vi "GUI_Cameras_TCP.vi"() -> ()   [LabVIEW 2013]
uses:
  <vilib>/Utility/tcp.llb/UDP Multicast Write-Only Open.vi
  <vilib>/Utility/file.llb/Read From Spreadsheet File (string).vi
  <vilib>/vision/Image Controls.llb/IMAQ Image.ctl
panel:
  out "New Image 2":T1
  in  "Device Name for vi mode":string="FakeCam1"
  out "x-y 2":u32(graph)
  out "x-y":i32(graph)
  out "x = y?":bool
  out "Numeric":i32
  out "#shot":i32=8
  out "x-y":u32(graph)
  out "data out 2":string
  out "Device Name":string="FakeCam1"
  in  "Device shotnumber":i32
  in  "New Shot":bool
  out "con ref array":refnum<vi>[](array[refnum])
  out "MC Multicast":refnum<k16>
  out "new Slow Data":bool
  out "new Device Data":bool
  in  "Tab Control":T2(tab)
  in  "setTrigger":bool
  in  "String":string="ScanStart>>Cam1only.txt"
  in  "send":bool
  in  "setSave":bool
  out "save":bool
  in  "setExposure":dbl=0.32000000000000006
  out "exposure":dbl=0.32
  out "trigger":bool=TRUE
  out "gain":dbl=10.0
  in  "setGain":dbl
  out "error message":string
  out "error":bool
  out "data out":string="Cam1>>ScanStart>>no error,>>"
  out "New Image":T1(plugin-control)
  in  "reset":bool
  in  "ScanEnd":bool
  in  "ScanStart":bool
  out "local Port":u16=64444
  out "Remote Host":string="192.168.10.157"
  out "port or service name":u16=65400
  in  "timeout ms (100)":i32=500
  in  "Multicast":bool=TRUE
  out "image \nconnection":bool
  out "data\nconnection":bool
  out "image con closed":bool=TRUE
  out "data con closed":bool=TRUE
  out "fast ID":refnum<k16>
  out "slow ID":refnum<k16>
  out "error out":errorcluster
  out "image connection ID":refnum<k5>
  out "data connection ID":refnum<k5>
  out "connections":variant[](array[variant])=[variant(refnum<k16> refnum), variant(refnum<k16> refnum)]
  in  "time to wait":i32=10
  in  "milliseconds to wait":u32=25
  in  "Image Subscriber list":string="wait>>image"
  in  "Subscriber list 2":string="wait>>exposure,trigger,save,gain"
  in  "Data String":string="exposure,0.320000\r\ntrigger,on\r\nsave,off\r\ngain,10.000000\r\n"
  out "Image":u8[][](graph)
  out "all rows":string[][](array[string])=[["localport", "64444"], ["port", "65400"], ["remotehost", "192.168.10.157"]]
  out "path":path=path "X:/Software/LOASIS Control System/Developers Version/Interface/GUI_Cameras/192.168.10.153.txt"
  out "My IP":string="192.168.10.153"
  in  "stop":bool
  # "61525"
  # "65535"
  # "61533"
  # "localhost"
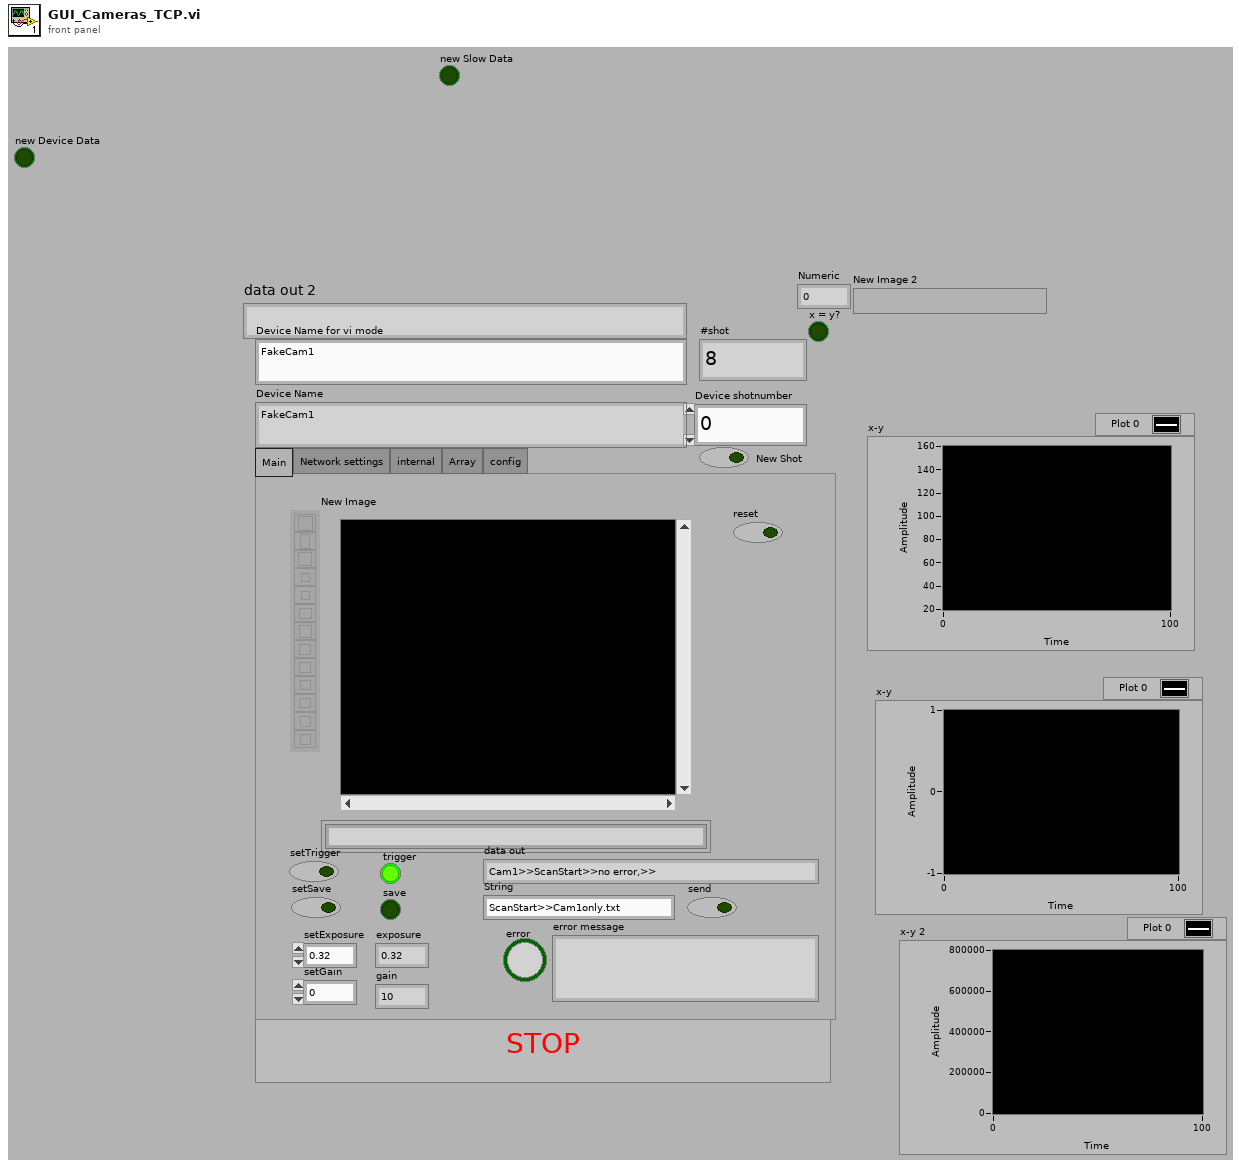
[diagram p1: front panel]
types:
  T1 = typedef "IMAQ Image.ctl" = refnum<image>
  T2 = enum32{"Main", "Network settings", "internal", "Array", "config"}
  T3 = typedef "Image Type" = u32
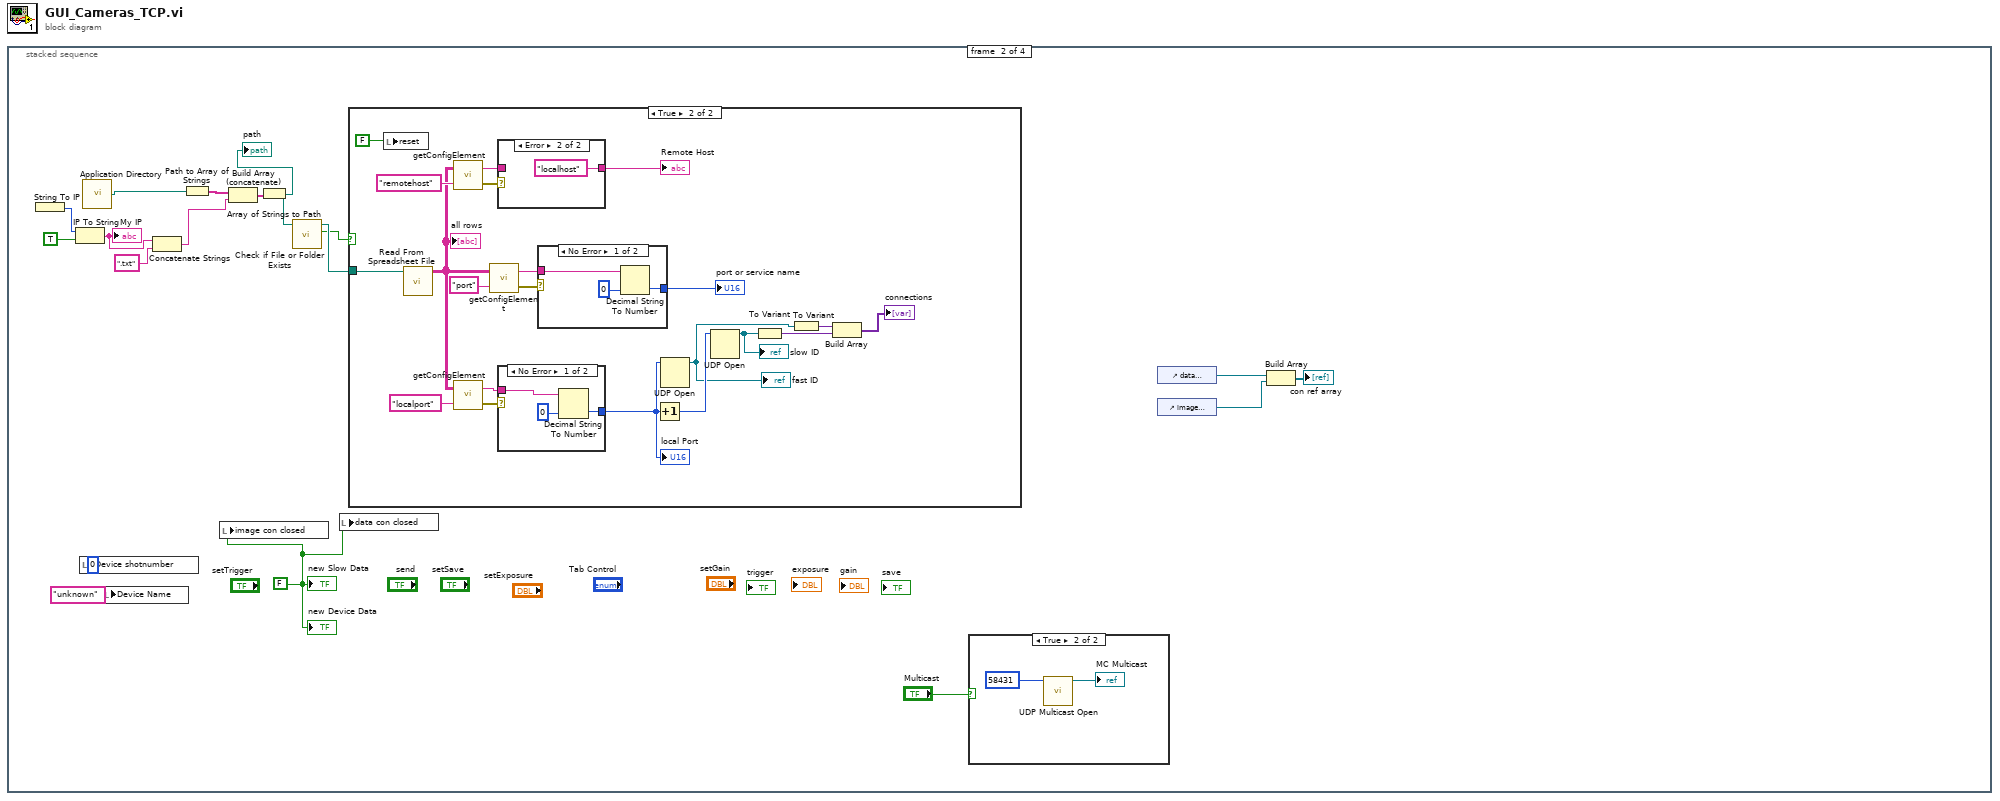
[diagram p0: block diagram]
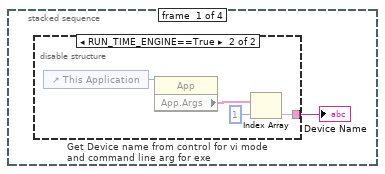
[diagram p2: hidden frame]
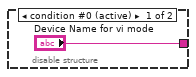
[diagram p3: hidden frame]
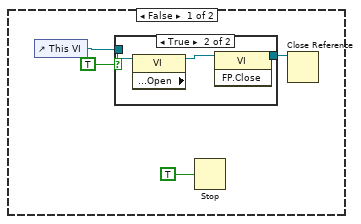
[diagram p4: hidden frame]
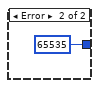
[diagram p6: hidden frame]
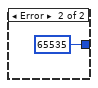
[diagram p8: hidden frame]
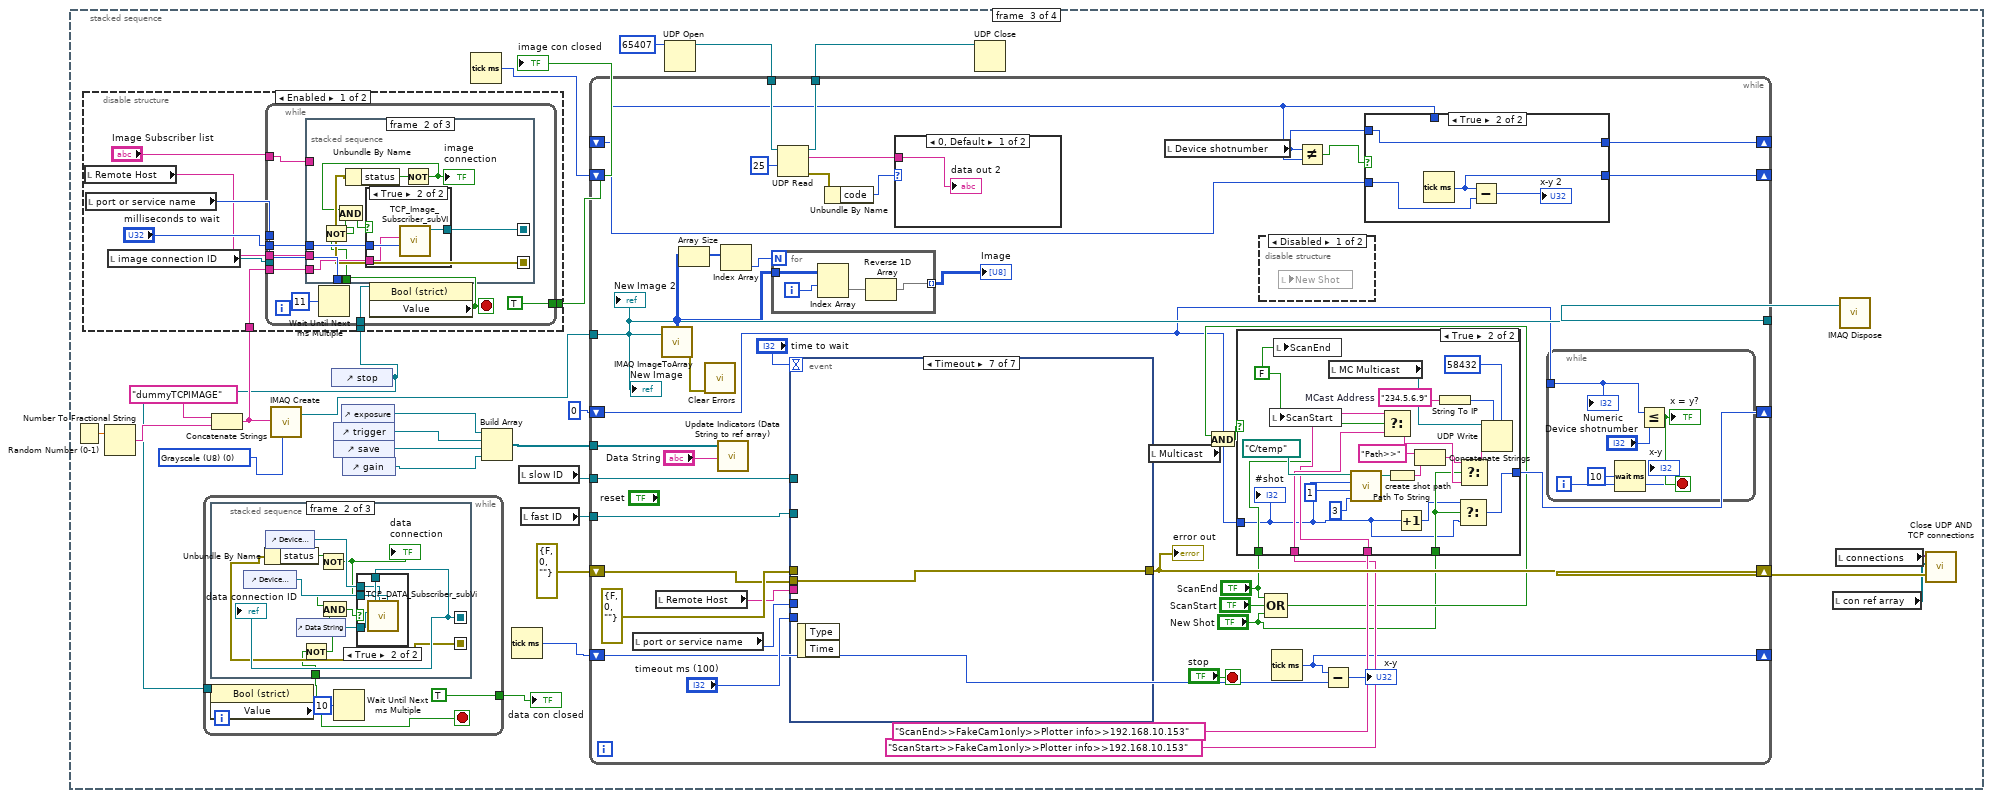
[diagram p10: hidden frame]
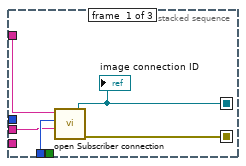
[diagram p11: hidden frame]
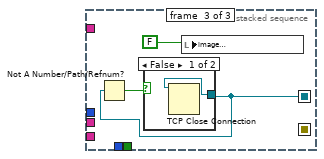
[diagram p13: hidden frame]
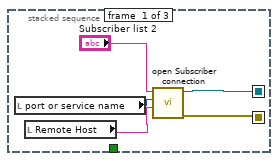
[diagram p16: hidden frame]
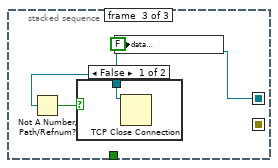
[diagram p18: hidden frame]
diagram:
  n1 = stacked-sequence {
    frame #0 {
      n2 = disable-structure "Get Device name from control for vi mode\nand command line arg for exe" shown="RUN_TIME_ENGINE==True" {
        disable-tunnel: ["Device Name for vi mode" w3] -> w1
        frame condition #0 (active) {
        }
        frame condition #1 {
          n3 = control-ref of="This Application"() -> (w6:refnum<vi>)
          n4 = property class="App"(reference=w6) -> ("App.Args"=w5:string[])  [unwired: 1 in, 2 out]
          n5 = Index Array(array=w5, index=1) -> (element=w3:string)
        }
      }
      "Device Name" <- w1
    }
    frame #1 {
      w7 = FALSE ("new Device Data")
      n6 = String To IP() -> (0:w16:u32)  [unwired: 1 in]
      n7 = IP To String(1:TRUE ("dot notation? (F)"), 2:w16) -> (0:w14:string)
      "My IP" <- w14
      n8 = local write "Device shotnumber"(0 ("shotnumber")) -> ()
      n9 = call <vilib>:"Application Directory.vi"() -> ("Application Directory"=w12:path)
      n10 = local write "Device Name"("unknown" ("Device Name")) -> ()
      n11 = Concatenate Strings(w14, ".txt" ("pattern")) -> (w11:string)
      n12 = Path to Array of Strings(0:w12) -> (2:w18:string[])  [unwired: 1 out]
      n13 = local write "image con closed"(w7) -> ()
      n14 = Build Array (concatenate)(w18, w11) -> (w17:string[])
      n15 = Array of Strings to Path(0:w17) -> (2:w10:path)  [unwired: 1 in]
      "path" <- w10
      n16 = call <vilib>:"Check if File or Folder Exists.vi"("path"=w10) -> ("file or folder exists?"=w8:bool, "dup path"=w9:path)  [unwired: 8 in, 1 out]
      n17 = local write "data con closed"(w7) -> ()
      n18 = case shown="True" w8 {
        tunnel: w9 -> [_ w33]
        frame False {
          n19 = control-ref of="This VI"() -> (w27:refnum<vi>)
          n20 = case shown="True" TRUE {
            tunnel: w27 -> [w29 w32]
            tunnel: [w29 w30] -> w26
            frame False {
            }
            frame True {
              n21 = property class="VI" props=["Front Panel.Open"](reference=w32) -> (reference out=w31:refnum<vi>)  [unwired: 1 in, 2 out]
              n22 = invoke class="VI" method="FP.Close"(reference=w31) -> (reference out=w30:refnum<vi>)  [unwired: 2 in, 2 out]
            }
          }
          n23 = Stop(stop? (T)=TRUE) -> ()
          n24 = Close Reference(reference=w26) -> ()  [unwired: 1 in, 1 out]
        }
        frame True {
          n25 = local write "reset"(FALSE ("reset")) -> ()
          n26 = call-poly <vilib>:"Read From Spreadsheet File.vi"("file path (dialog if empty)"=w33) -> ("all rows"=w35:string[][])  [unwired: 6 in, 4 out]
          "all rows" <- w35
          n27 = call "getConfigElement.vi"("element"="remotehost", "all rows"=w35) -> ("error in"=w42:errorcluster, "value"=w41:string)
          n28 = call "getConfigElement.vi"("element"="localport", "all rows"=w35) -> ("error in"=w44:errorcluster, "value"=w45:string)
          n29 = call "getConfigElement.vi"("element"="port", "all rows"=w35) -> ("error in"=w38:errorcluster, "value"=w37:string)
          n30 = case shown="Error" w42 {
            tunnel: w41 -> [w58 _]
            tunnel: [w58 "localhost" ("value")] -> w39
            frame No Error {
            }
            frame Error {
            }
          }
          "Remote Host" <- w39
          n31 = case shown="No Error" w44 {
            tunnel: w45 -> [w62 _]
            tunnel: [w60 u16 65535] -> w43
            frame No Error {
              n32 = Decimal String To Number(string=w62, default (0L)=u16 0 ("local Port")) -> (number=w60:u16)  [unwired: 1 in, 1 out]
            }
            frame Error {
            }
          }
          "local Port" <- w43
          n33 = case shown="No Error" w38 {
            tunnel: w37 -> [w56 _]
            tunnel: [w54 u16 65535] -> w34
            frame No Error {
              n34 = Decimal String To Number(string=w56, default (0L)=u16 0 ("local Port")) -> (number=w54:u16)  [unwired: 1 in, 1 out]
            }
            frame Error {
            }
          }
          "port or service name" <- w34
          n35 = Increment(x=w43) -> (x+1=w53:u16)
          n36 = UDP Open(11:w43) -> (port=w51:refnum<k16>)  [unwired: 4 in, 2 out]
          "fast ID" <- w51
          n37 = UDP Open(11:w53) -> (port=w50:refnum<k16>)  [unwired: 4 in, 2 out]
          "slow ID" <- w50
          n38 = To Variant(anything=w50) -> (Variant=w48:variant)
          n39 = To Variant(anything=w51) -> (Variant=w49:variant)
          n40 = Build Array(w49, w48) -> (→"connections":variant[])
        }
      }
      n41 = case shown="True" "Multicast" {
        frame False {
        }
        frame True {
          n42 = call-poly <vilib>:"UDP Multicast Open.vi"("port"=u16 58431) -> ("connection ID"=→"MC Multicast":refnum<k16>)  [unwired: 9 in, 1 out]
        }
      }
      n43 = control-ref of="data connection ID"() -> (w24:refnum<vi>)
      n44 = control-ref of="image connection ID"() -> (w23:refnum<vi>)
      n45 = Build Array(w24, w23) -> (→"con ref array":refnum<vi>[])
      "new Device Data" <- w7
      "new Slow Data" <- w7
    }
    frame #2 {
      w86 = T3 0 items=["Grayscale (U8)", "Grayscale (I16)", "Grayscale (SGL)", "Complex (CSG)", "RGB (U32)", "HSL (U32)", "RGB (U64)", "Grayscale (U16)"] ("Image Type")
      n46 = Random Number (0-1)() -> (number: 0 to 1=w83:dbl)
      n47 = Number To Fractional String(number=w83) -> (F-format string=w82:string)  [unwired: 3 in]
      n48 = Concatenate Strings("dummyTCPIMAGE" ("Image Name"), w82) -> (w80:string)
      n49 = call "IMAQ Create"("Image Name"=w80, "Image Type"=w86) -> ("New Image"=w85:T1)  [unwired: 3 in, 1 out]
      n50 = control-ref of="stop"() -> (w73:refnum<vi>)
      n51 = disable-structure shown="Enabled" {
        disable-tunnel: w80 -> [w98 _]
        disable-tunnel: [w94 _] -> w75
        disable-tunnel: w73 -> [w93 _]
        frame Enabled {
          n52 = local read "Remote Host"() -> (w96:string)
          n53 = local read "port or service name"() -> (w97:u16)
          n54 = local read "image connection ID"() -> (w100:refnum<k5>)
          n55 = while {
            tunnel: w100 -> [_]
            tunnel: "milliseconds to wait" -> [w109]
            tunnel: w98 -> [w108]
            tunnel: w97 -> [w107]
            tunnel: w96 -> [w106]
            tunnel: "Image Subscriber list" -> [w105]
            tunnel: [TRUE] -> w94
            tunnel: w93 -> [w102]
            stop <- w101 stop-if-true
            n56 = Wait Until Next ms Multiple(millisecond multiple=u32 11) -> ()  [unwired: 1 out]
            n57 = property class="Bool (strict)"(reference=w102) -> ("Value"=w101:bool)  [unwired: 1 in, 2 out]
            n58 = stacked-sequence {
              seq-local: [w112 _ _] -> [_ w121 w128]
              seq-local: [w110 _ _] -> [_ w120 _]
              tunnel: w109 -> [_ w123 _]
              tunnel: w108 -> [_ w122 _]
              tunnel: w107 -> [w114 _ _]
              tunnel: w106 -> [w113 _ _]
              tunnel: w105 -> [w111 _ _]
              tunnel: w101 -> [_ w118 _]
              frame #0 {
                n59 = call "open Subscriber connection.vi"("Machine"=w113, "Port"=w114, "Subscriber list"=w111) -> ("error out"=w110:errorcluster, "connection ID"=w112:refnum<k5>)  [unwired: 3 in]
                "image connection ID" <- w112
              }
              frame #1 {
                n60 = Not(x=w118) -> (.not. x?=w117:bool)
                n61 = Unbundle By Name(w120) -> ("status"=w119:bool)
                n62 = Not(x=w119) -> (.not. x?=w116:bool)
                "image \nconnection" <- w116
                n63 = And(x=w116, y=w117) -> (x .and. y?=w115:bool)
                n64 = case shown="True" w115 {
                  tunnel: w123 -> [_ w126]
                  tunnel: w122 -> [_ w125]
                  tunnel: w121 -> [_ w124]
                  frame False {
                  }
                  frame True {
                    n65 = call "TCP_Image_Subscriber_subVI.vi"(9:w126, "Image Name"=w125, "connection ID"=w124) -> ()  [unwired: 8 in, 1 out]
                  }
                }
              }
              frame #2 {
                n66 = Not A Number/Path/Refnum?(number/path/refnum=w128) -> (NaN/Path/Refnum?=w129:bool)
                n67 = case shown="False" w129 {
                  tunnel: w128 -> [w130 _]
                  frame False {
                    n68 = TCP Close Connection(connection ID=w130) -> ()  [unwired: 2 in, 2 out]
                  }
                  frame True {
                  }
                }
                n69 = local write "image \nconnection"(FALSE ("status")) -> ()
              }
            }
          }
        }
        frame Disabled {
        }
      }
      "image con closed" <- w75
      n70 = while {
        tunnel: [TRUE] -> w74
        tunnel: w73 -> [w132]
        stop <- w131 stop-if-true
        n71 = property class="Bool (strict)"(reference=w132) -> ("Value"=w131:bool)  [unwired: 1 in, 2 out]
        n72 = stacked-sequence {
          seq-local: [w136 _ _] -> [_ w148 w155]
          seq-local: [w135 _ _] -> [_ w147 _]
          tunnel: w131 -> [_ w141 _]
          frame #0 {
            n73 = local read "port or service name"() -> (w138:u16)
            n74 = local read "Remote Host"() -> (w137:string)
            n75 = call "open Subscriber connection.vi"("Machine"=w137, "Port"=w138, "Subscriber list"="Subscriber list 2") -> ("error out"=w135:errorcluster, "connection ID"=w136:refnum<k5>)  [unwired: 3 in]
          }
          frame #1 {
            n76 = control-ref of="Device shotnumber"() -> (w146:refnum<vi>)
            n77 = Unbundle By Name(w147) -> ("status"=w144:bool)
            n78 = control-ref of="Device Name"() -> (w145:refnum<vi>)
            n79 = control-ref of="Data String"() -> (w149:refnum<vi>)
            n80 = Not(x=w141) -> (.not. x?=w142:bool)
            n81 = Not(x=w144) -> (.not. x?=w143:bool)
            "data\nconnection" <- w143
            n82 = And(x=w143, y=w142) -> (x .and. y?=w140:bool)
            n83 = case shown="True" w140 {
              tunnel: w149 -> [_ w153]
              tunnel: w148 -> [_ w152]
              tunnel: w146 -> [_ w151]
              tunnel: w145 -> [_ w150]
              frame False {
              }
              frame True {
                n84 = call "TCP_DATA_Subscriber_subVi.vi"("shot number"=w151, "whatamI"=w150, 10:w153, "connection ID"=w152) -> ()  [unwired: 7 in, 1 out]
              }
            }
            "data connection ID" <- w148
          }
          frame #2 {
            n85 = Not A Number/Path/Refnum?(number/path/refnum=w155) -> (NaN/Path/Refnum?=w156:bool)
            n86 = case shown="False" w156 {
              tunnel: w155 -> [w157 _]
              frame False {
                n87 = TCP Close Connection(connection ID=w157) -> ()  [unwired: 2 in, 2 out]
              }
              frame True {
              }
            }
            n88 = local write "data\nconnection"(FALSE ("status 2")) -> ()
          }
        }
        n89 = Wait Until Next ms Multiple(millisecond multiple=u32 10) -> ()  [unwired: 1 out]
      }
      "data con closed" <- w74
      n90 = control-ref of="trigger"() -> (w87:refnum<vi>)
      n91 = control-ref of="save"() -> (w71:refnum<vi>)
      n92 = control-ref of="exposure"() -> (w88:refnum<vi>)
      n93 = control-ref of="gain"() -> (w72:refnum<vi>)
      n94 = Tick Count (ms)() -> (millisecond timer value=w66:u32)
      n95 = Build Array(w88, w87, w71, w72) -> (w79:refnum<vi>[])
      n96 = Tick Count (ms)() -> (millisecond timer value=w67:u32)
      n97 = local read "slow ID"() -> (w90:refnum<k16>)
      n98 = local read "fast ID"() -> (w91:refnum<k16>)
      n99 = UDP Open(11:u16 65407 ("port")) -> (port=w69:refnum<k16>)  [unwired: 4 in, 2 out]
      n100 = while {
        tunnel: w91 -> [w191]
        shift-right: [w189] -> w84
        shift-left: errorcluster {"status"=FALSE, "code"=0, "source"=""} ("error out") -> [w195]
        tunnel: w90 -> [w185]
        tunnel: w85 -> [w198]
        tunnel: [w198] -> w89
        tunnel: w79 -> [w197]
        shift-right: [w188] -> _
        shift-left: 0 -> [w164]
        tunnel: w69 -> [w178]
        tunnel: [w177] -> w68
        shift-right: [w166] -> _
        shift-left: w67 -> [w167]
        shift-right: [w161] -> _
        shift-left: _ -> [w158]
        shift-right: [w159] -> _
        shift-left: w66 -> [w160]
        stop <- "stop" stop-if-true
        n101 = local read "port or service name"() -> (w192:u16)
        n102 = local read "Remote Host"() -> (w193:string)
        n103 = call "IMAQ ImageToArray"("Image"=w198) -> ("error out"=w184:errorcluster, "Image Pixels (U8)"=w181:u8[][])  [unwired: 3 in, 3 out]
        n104 = Array Size(array=w181) -> (size(s)=w183:i32[])
        n105 = call <vilib>:"Clear Errors.vi"("error in (no error)"=w184) -> ()  [unwired: 6 in, 1 out]
        n106 = call "Update Indicators (Data String to ref array).vi"("Data String"="Data String", "Array"=w197) -> ()  [unwired: 4 in]
        n107 = Index Array(array=w183) -> (element=w182:i32)  [unwired: 1 in]
        n108 = for {
          N: w182 -> [_]
          tunnel: w181 -> [w216]
          tunnel: [w214] -> w180 mode=indexing
          i -> [w213]
          n109 = Index Array(array=w216, index (row)=w213) -> (element=w215:u8[])  [unwired: 1 in]
          n110 = Reverse 1D Array(array=w215) -> (reversed array=w214:u8[])
        }
        "Image" <- w180
        n111 = UDP Read(connection ID=w178, timeout ms (25000)=25) -> (data out=w173:string, error out=w175:errorcluster, 3:w177:refnum<k16>)  [unwired: 2 in, 2 out]
        n112 = event shown="[6] Timeout" {
          selector: _ -> [_ _ _ _ _ _ _]
          dyn-events: _ -> [_ _ _ _ _ _ _]
          timeout: "time to wait" -> [_ _ _ _ _ _ _]
          tunnel: w191 -> [w243 w261 _ w277 w290 w306 _]
          tunnel: [w241 w259 _ w275 w287 w304 w310] -> w189
          tunnel: errorcluster {"status"=FALSE, "code"=0, "source"=""} ("error out") -> [w242 w260 _ w276 w288 w305 _]
          tunnel: w193 -> [w246 w258 _ w274 w291 w303 _]
          tunnel: w192 -> [w247 w257 _ w273 w286 w302 _]
          tunnel: "timeout ms (100)" -> [w248 w256 _ w272 w285 w301 _]
          tunnel: w185 -> [w244 w262 _ w278 w289 w307 _]
          tunnel: w195 -> [_ _ _ _ _ _ w310]
          event "setTrigger": Value Change {
            n113 = event-data() -> ("NewVal"=w253:bool)  [unwired: 1 in, 4 out]
            n114 = Select(t="on", s=w253, f="off") -> (s? t:f=w249:string)
            n115 = Concatenate Strings("settrigger>>" ("data in"), w249) -> (w245:string)
            n116 = call "sendCommandAndListen.vi"(0:w244, 1:w243, "command in"=w245, "error in"=w242, "Remote Host"=w246, "port or service name"=w247, "timeout ms (100)"=w248) -> ("error"=w239:bool, "error message"=w240:string, "error out"=w241:errorcluster)  [unwired: 5 in, 5 out]
            n117 = local write "error message"(w240) -> ()
            n118 = local write "error"(w239) -> ()
          }
          event "setExposure": Value Change {
            n119 = event-data() -> ("NewVal"=w264:dbl)  [unwired: 1 in, 4 out]
            n120 = Number To Fractional String(number=w264) -> (F-format string=w265:string)  [unwired: 3 in]
            n121 = Concatenate Strings("setexposure>>" ("data in"), w265) -> (w263:string)
            n122 = call "sendCommandAndListen.vi"(0:w262, 1:w261, "command in"=w263, "error in"=w260, "Remote Host"=w258, "port or service name"=w257, "timeout ms (100)"=w256) -> ("error"=→"error":bool, "error message"=→"error message":string, "error out"=w259:errorcluster)  [unwired: 5 in, 5 out]
          }
          event "reset": Value Change {
            n123 = event-data() -> ()  [unwired: 1 in, 5 out]
            n124 = local read "con ref array"() -> (w268:refnum<vi>[])
            n125 = local write "Device Name"("unknown" ("Device Name")) -> ()
            n126 = local write "reset"(FALSE ("reset")) -> ()
            n127 = call "Close UDP AND TCP connections.vi"("appended array 2"=w268) -> ()  [unwired: 7 in]
          }
          event "setGain": Value Change {
            n128 = event-data() -> ("NewVal"=w280:dbl)  [unwired: 1 in, 4 out]
            n129 = Number To Fractional String(number=w280) -> (F-format string=w281:string)  [unwired: 3 in]
            n130 = Concatenate Strings("setgain>>" ("data in"), w281) -> (w279:string)
            n131 = call "sendCommandAndListen.vi"(0:w278, 1:w277, "command in"=w279, "error in"=w276, "Remote Host"=w274, "port or service name"=w273, "timeout ms (100)"=w272) -> ("error"=w270:bool, "error message"=w271:string, "error out"=w275:errorcluster)  [unwired: 5 in, 5 out]
            n132 = local write "error message"(w271) -> ()
            n133 = local write "error"(w270) -> ()
          }
          event "setSave": Value Change {
            n134 = event-data() -> ("NewVal"=w297:bool)  [unwired: 1 in, 4 out]
            n135 = Select(t="on", s=w297, f="off") -> (s? t:f=w293:string)
            n136 = Concatenate Strings("setsave>>" ("data in"), w293) -> (w292:string)
            n137 = call "sendCommandAndListen.vi"(0:w289, 1:w290, "command in"=w292, "error in"=w288, "Remote Host"=w291, "port or service name"=w286, "timeout ms (100)"=w285) -> ("error"=w283:bool, "error message"=w284:string, "error out"=w287:errorcluster)  [unwired: 5 in, 5 out]
            n138 = local write "error message"(w284) -> ()
            n139 = local write "error"(w283) -> ()
          }
          event "send": Value Change {
            n140 = event-data() -> ()  [unwired: 1 in, 5 out]
            n141 = local write "send"(FALSE ("sent")) -> ()
            n142 = call "sendCommandAndListen.vi"(0:w307, 1:w306, "command in"="String", "error in"=w305, "Remote Host"=w303, "port or service name"=w302, "timeout ms (100)"=w301) -> ("error"=w299:bool, "error message"=w300:string, "data out"=→"data out":string, "error out"=w304:errorcluster)  [unwired: 5 in, 4 out]
            n143 = local write "error message"(w300) -> ()
            n144 = local write "error"(w299) -> ()
          }
          event Timeout {
            n145 = event-data() -> ()  [unwired: 1 in, 2 out]
          }
        }
        "error out" <- w189
        n146 = Unbundle By Name(w175) -> ("code"=w174:i32)
        n147 = case shown="0, Default" w174 {
          tunnel: w173 -> [w212 _]
          frame 0, Default {
            "data out 2" <- w212
          }
          frame 56 {
          }
        }
        n148 = local read "Multicast"() -> (w187:bool)
        n149 = local read "Device shotnumber"() -> (w162:i32)
        n150 = disable-structure shown="Disabled" {
          frame Disabled {
            n151 = local read "New Shot"() -> ()  [unwired: 1 in]
          }
          frame Enabled {
          }
        }
        n152 = Compound Arithmetic op=OR("ScanEnd", "ScanStart", "New Shot") -> (w170:bool)
        n153 = And(x=w170, y=w187) -> (x .and. y?=w186:bool)
        n154 = case shown="True" w186 {
          tunnel: w164 -> [w217 w219]
          tunnel: [w217 w218] -> w188
          tunnel: "New Shot" -> [_ w221]
          tunnel: "ScanEnd>>FakeCam1only>>Plotter info>>192.168.10.153" ("String 2") -> [_ w226]
          tunnel: "ScanStart>>FakeCam1only>>Plotter info>>192.168.10.153" ("String 3") -> [_ w227]
          tunnel: "ScanEnd" -> [_ w223]
          frame False {
          }
          frame True {
            w222 = FALSE ("New Shot")
            w232 = "234.5.6.9"  # MCast Address
            n155 = local write "ScanStart"(w222) -> ()
            n156 = local write "ScanEnd"(w222) -> ()
            n157 = local read "MC Multicast"() -> (w233:refnum<k16>)
            n158 = call "create shot path.vi"("width (-)"=i16 3, "Shot Number"=w219, "Scan Number"=1, "Scans Path"=path "C:/temp") -> ("Device xxx path"=w236:path)  [unwired: 2 in]
            n159 = Select(t=w226, s=w223, f=w227) -> (s? t:f=w225:string)
            n160 = Path To String(path=w236) -> (string=w234:string)
            n161 = Increment(x=w219) -> (x+1=w220:i32)
            n162 = Concatenate Strings("Path>>" ("string"), w234) -> (w224:string)
            n163 = String To IP(1:w232) -> (0:w238:u32)
            n164 = Select(t=w220, s=w221, f=w219) -> (s? t:f=w218:i32)
            n165 = Select(t=w224, s=w221, f=w225) -> (s? t:f=w228:string)
            n166 = UDP Write(address=w238, port or service name=u16 58432, connection ID=w233, data in=w228) -> ()  [unwired: 2 in, 2 out]
            "#shot" <- w219
          }
        }
        n167 = Tick Count (ms)() -> (millisecond timer value=w166:u32)
        n168 = Not Equal?(x=w162, y=w158) -> (x != y?=w163:bool)
        n169 = Subtract(x=w166, y=w167) -> (x-y=→"x-y":u32)
        n170 = case shown="True" w163 {
          tunnel: w162 -> [_ w206]
          tunnel: [w202 w206] -> w161
          tunnel: w158 -> [w202 _]
          tunnel: w160 -> [w201 w205]
          tunnel: [w201 w204] -> w159
          frame False {
          }
          frame True {
            n171 = Tick Count (ms)() -> (millisecond timer value=w204:u32)
            n172 = Subtract(x=w204, y=w205) -> (x-y=→"x-y 2":u32)
          }
        }
        n173 = while {
          tunnel: w164 -> [w210]
          i -> [w207]
          stop <- w208 stop-if-true
          n174 = Wait (ms)(milliseconds to wait=u32 10) -> ()  [unwired: 1 out]
          n175 = Less Or Equal?(x=w210, y="Device shotnumber") -> (x <= y?=w208:bool)
          "x = y?" <- w208
          "Numeric" <- w210
          "x-y" <- w207
        }
        "New Image" <- w198
        "New Image 2" <- w198
      }
      n176 = UDP Close(connection ID=w68) -> ()  [unwired: 1 in, 2 out]
      n177 = local read "con ref array"() -> (w78:refnum<vi>[])
      n178 = local read "connections"() -> (w76:variant[])
      n179 = call "IMAQ Dispose"("Image"=w89) -> ()  [unwired: 5 in, 1 out]
      n180 = call "Close UDP AND TCP connections.vi"("error in"=w84, "appended array 2"=w78, "appended array"=w76) -> ()  [unwired: 5 in]
    }
    frame #3 {
      n181 = flat-sequence {
        frame #0 {
          n182 = Wait (ms)(milliseconds to wait=u32 0) -> ()  [unwired: 1 out]
        }
        frame #1 {
          n183 = local write "stop"(FALSE ("stop")) -> ()
        }
        frame #2 {
          n184 = control-ref of="This VI"() -> (w315:refnum<vi>)
          n185 = case shown="True" FALSE {
            tunnel: w315 -> [w316 w319]
            tunnel: [w316 w317] -> w314
            frame False {
            }
            frame True {
              n186 = property class="VI" props=["Front Panel.Open"](reference=w319) -> (reference out=w318:refnum<vi>)  [unwired: 1 in, 2 out]
              n187 = invoke class="VI" method="FP.Close"(reference=w318) -> (reference out=w317:refnum<vi>)  [unwired: 2 in, 2 out]
            }
          }
          n188 = Close Reference(reference=w314) -> ()  [unwired: 1 in, 1 out]
        }
      }
    }
  }
